vi "SplineHelp_ThomasAlgorithm.vi"(6 "inputSolutionVector":dbl[](array[numeric]), 8 "D":dbl[](array[numeric]), 9 "C":dbl[](array[numeric]), 10 "B":dbl[](array[numeric]), 11 "A":dbl[](array[numeric])) -> (0 "error out":errorcluster, 3 "SolutionVector":dbl[](array[numeric]))   [LabVIEW 2019, in "Trajectory_Library.lvlib"]
doc: "Thomas algorithm for solving tridiagonal systems Af = d.\n \nParameters:\n - a - the values of A above the diagonal\n - b - the values of A on the diagonal\n - c - the values of A below the diagonal\n - d - the vector on the rhs\n - InputSolutionVector - the unknown (solution) vector\n\nReturns:\n - SolutionVector - The modifed solution vector\n - Error Out - Returned error cluster"
uses:
  Trajectory_Library.lvlib
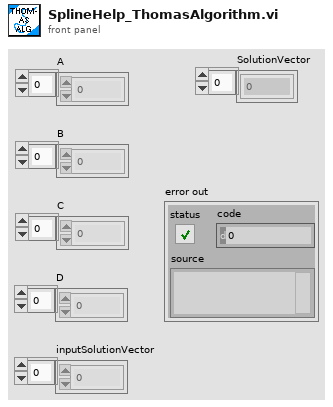
[diagram p1: front panel]
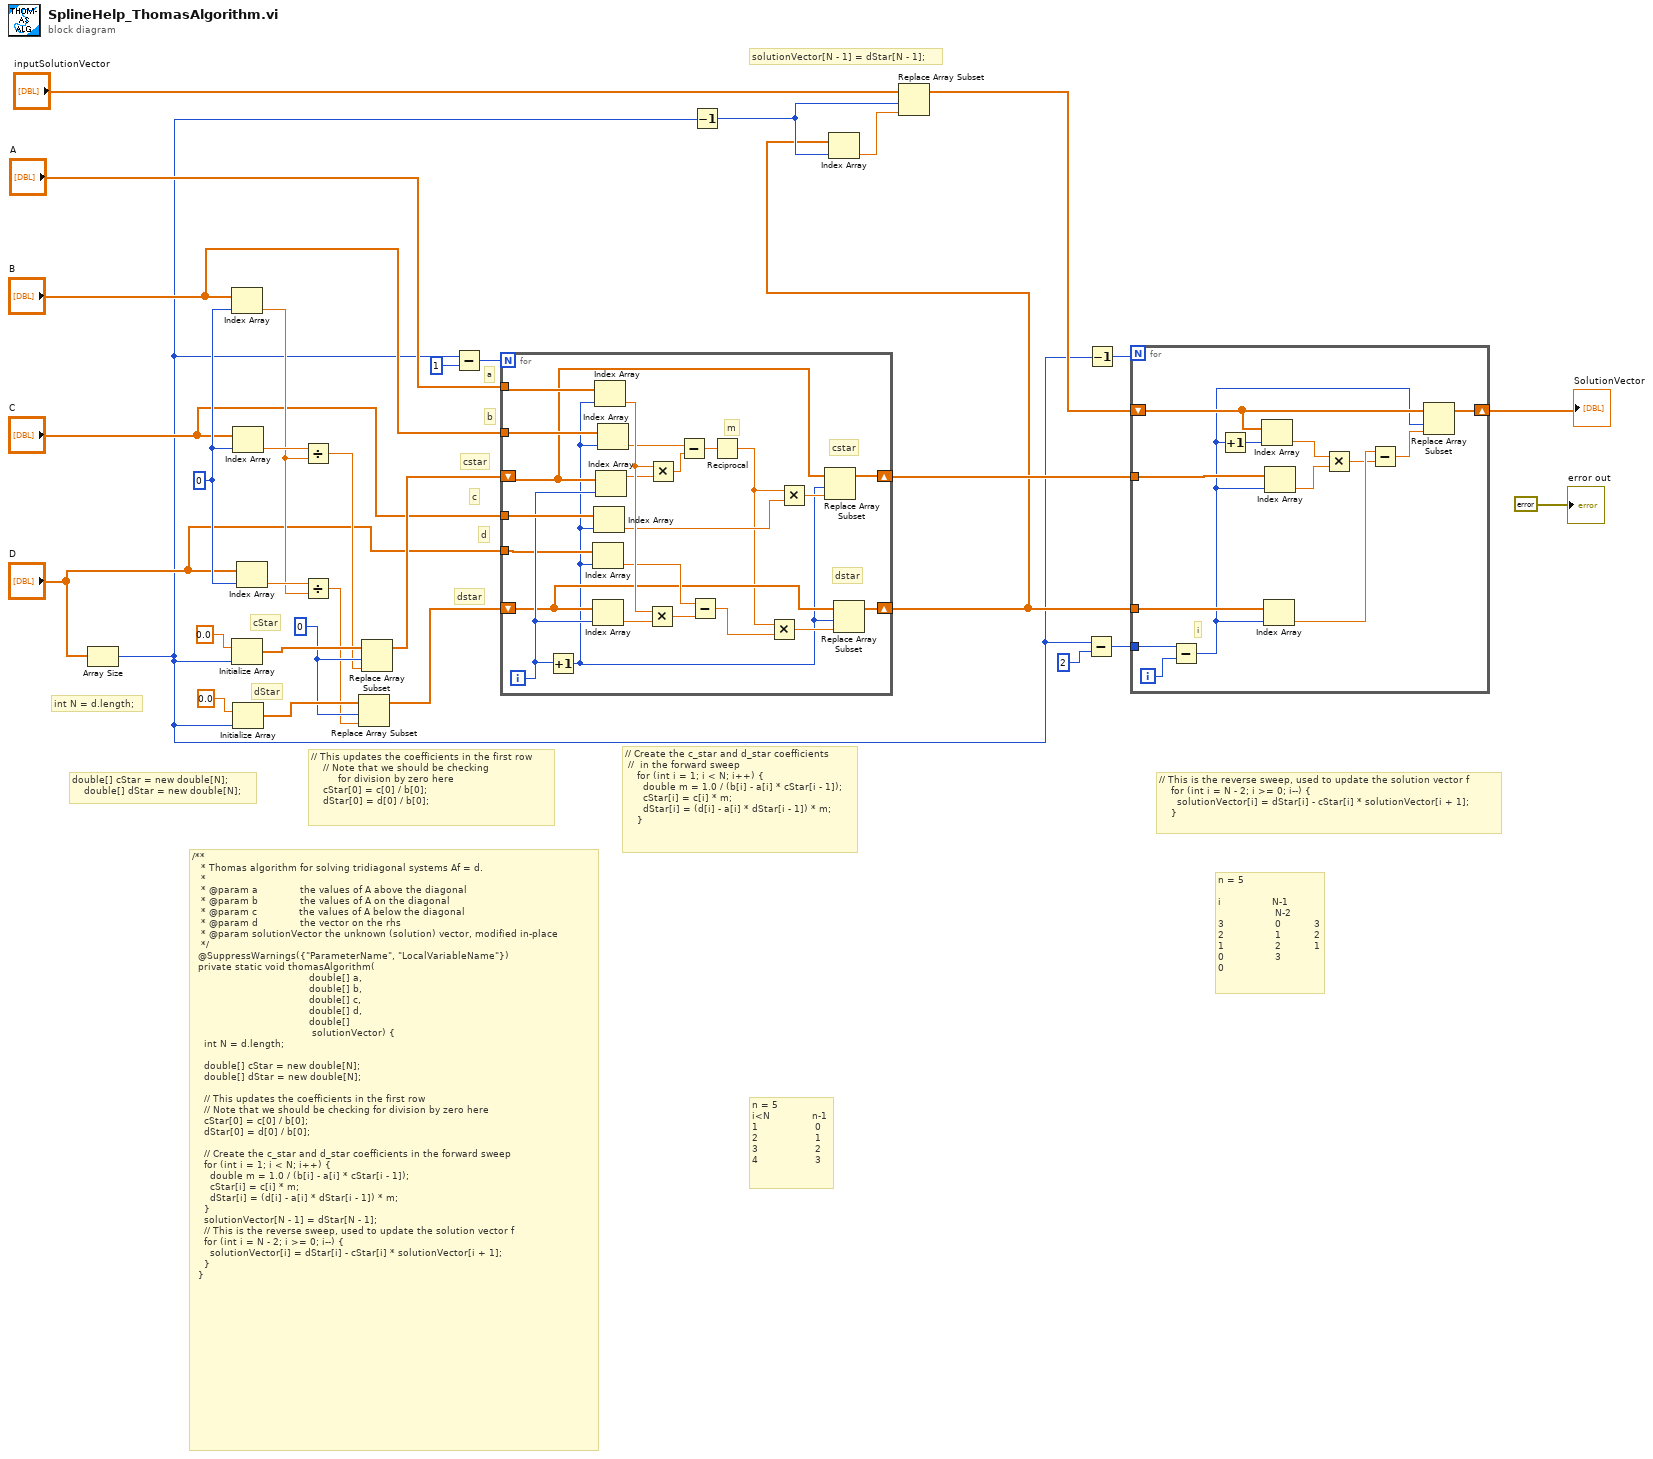
[diagram p0: block diagram]
diagram:
  w23 = 0 ("index")
  w29 = 0 ("index")
  # "n = 5\n\ni                 N-1\n                   N-2    \n3                 0           3\n2                 1           2\n1                 2           1\n0                 3            0"
  # "n = 5\ni<N              n-1\n1                   0\n2                   1\n3                   2\n4                   3"
  # "// This is the reverse sweep, used to update the solution vector f\n    for (int i = N - 2; i >= 0; i--) {\n      solutionVector[i] = dStar[i] - cStar[i] * solutionVector[i + 1];\n    }"
  # "solutionVector[N - 1] = dStar[N - 1];"
  # "d"
  # "dstar"
  # "c"
  # "cstar"
  # "b"
  # "a"
  # "// Create the c_star and d_star coefficients\n //  in the forward sweep\n    for (int i = 1; i < N; i++) {\n      double m = 1.0 / (b[i] - a[i] * cStar[i - 1]);\n      cStar[i] = c[i] * m;\n      dStar[i] = (d[i] - a[i] * dStar[i - 1]) * m;\n    }"
  # "// This updates the coefficients in the first row\n    // Note that we should be checking \n         for division by zero here\n    cStar[0] = c[0] / b[0];\n    dStar[0] = d[0] / b[0];"
  # "double[] cStar = new double[N];\n    double[] dStar = new double[N];"
  # "dStar"
  # "cStar"
  # "int N = d.length;"
  # "/**\n   * Thomas algorithm for solving tridiagonal systems Af = d.\n   *\n   * @param a              the values of A above the diagonal\n   * @param b              the values of A on the diagonal\n   * @param c              the values of A below the diagonal\n   * @param d              the vector on the rhs\n   * @param solutionVector the unknown (solution) vector, modified in-place\n   */\n  @SuppressWarnings({\"ParameterName\", \"LocalVariableName\"})\n  private static void thomasAlgorithm(\n                                       double[] a, \n                                       double[] b,\n                                       double[] c, \n                                       double[] d, \n                                       double[] \n                                        solutionVector) {\n    int N = d.length;\n\n    double[] cStar = new double[N];\n    double[] dStar = new double[N];\n\n    // This updates the coefficients in the first row\n    // Note that we should be checking for division by zero here\n    cStar[0] = c[0] / b[0];\n    dStar[0] = d[0] / b[0];\n\n    // Create the c_star and d_star coefficients in the forward sweep\n    for (int i = 1; i < N; i++) {\n      double m = 1.0 / (b[i] - a[i] * cStar[i - 1]);\n      cStar[i] = c[i] * m;\n      dStar[i] = (d[i] - a[i] * dStar[i - 1]) * m;\n    }\n    solutionVector[N - 1] = dStar[N - 1];\n    // This is the reverse sweep, used to update the solution vector f\n    for (int i = N - 2; i >= 0; i--) {\n      solutionVector[i] = dStar[i] - cStar[i] * solutionVector[i + 1];\n    }\n  }"
  n1 = Array Size(array="D") -> (size(s)=w2:i32)
  n2 = Index Array(array="B", index=w29) -> (element=w26:dbl)
  n3 = Initialize Array(0.0 ("element"), w2) -> (w25:dbl[])
  n4 = Index Array(array="C", index=w29) -> (element=w28:dbl)
  n5 = Initialize Array(0.0 ("element"), w2) -> (w24:dbl[])
  n6 = Index Array(array="D", index=w29) -> (element=w27:dbl)
  n7 = Divide(x=w28, y=w26) -> (x/y=w21:dbl)
  n8 = Divide(x=w27, y=w26) -> (x/y=w22:dbl)
  n9 = Replace Array Subset(array=w24, new element=w22, index=w23) -> (w18:dbl[])
  n10 = Replace Array Subset(array=w25, new element=w21, index=w23) -> (w19:dbl[])
  n11 = Subtract(x=w2, y=1) -> (x-y=w20:i32)
  n12 = for {
    N: w20 -> [_]
    tunnel: "A" -> [w54]
    tunnel: "B" -> [w52]
    tunnel: "C" -> [w49]
    shift-right: [w46] -> w7
    shift-left: w19 -> [w45]
    tunnel: "D" -> [w39]
    shift-right: [w36] -> w6
    shift-left: w18 -> [w35]
    i -> [w41]
    # "dstar"
    # "cstar"
    # "m"
    n13 = Increment(x=w41) -> (x+1=w32:i32)
    n14 = Index Array(array=w39, index=w32) -> (element=w38:dbl)
    n15 = Index Array(array=w35, index=w41) -> (element=w42:dbl)
    n16 = Index Array(array=w49, index=w32) -> (element=w43:dbl)
    n17 = Index Array(array=w54, index=w32) -> (element=w53:dbl)
    n18 = Index Array(array=w45, index=w41) -> (element=w47:dbl)
    n19 = Index Array(array=w52, index=w32) -> (element=w51:dbl)
    n20 = Multiply(x=w53, y=w42) -> (x*y=w40:dbl)
    n21 = Multiply(x=w53, y=w47) -> (x*y=w50:dbl)
    n22 = Subtract(x=w51, y=w50) -> (x-y=w48:dbl)
    n23 = Subtract(x=w38, y=w40) -> (x-y=w33:dbl)
    n24 = Reciprocal(x=w48) -> (1/x=w34:dbl)
    n25 = Multiply(x=w34, y=w33) -> (x*y=w37:dbl)
    n26 = Multiply(x=w34, y=w43) -> (x*y=w44:dbl)
    n27 = Replace Array Subset(array=w45, new element=w44, index=w32) -> (w46:dbl[])
    n28 = Replace Array Subset(array=w35, new element=w37, index=w32) -> (w36:dbl[])
  }
  n29 = Decrement(x=w2) -> (x-1=w12:i32)
  n30 = Index Array(array=w6, index=w12) -> (element=w11:dbl)
  n31 = Replace Array Subset(array="inputSolutionVector", new element=w11, index=w12) -> (w5:dbl[])
  n32 = Subtract(x=w2, y=2) -> (x-y=w9:i32)
  n33 = Decrement(x=w2) -> (x-1=w8:i32)
  n34 = for {
    N: w8 -> [_]
    tunnel: w9 -> [w66]
    tunnel: w7 -> [w64]
    tunnel: w6 -> [w63]
    shift-right: [w62] -> w4
    shift-left: w5 -> [w61]
    i -> [w67]
    # "i"
    n35 = Subtract(x=w66, y=w67) -> (x-y=w60:i32)
    n36 = Increment(x=w60) -> (x+1=w65:i32)
    n37 = Index Array(array=w61, index=w65) -> (element=w56:dbl)
    n38 = Index Array(array=w63, index=w60) -> (element=w58:dbl)
    n39 = Index Array(array=w64, index=w60) -> (element=w57:dbl)
    n40 = Multiply(x=w56, y=w57) -> (x*y=w55:dbl)
    n41 = Subtract(x=w58, y=w55) -> (x-y=w59:dbl)
    n42 = Replace Array Subset(array=w61, new element=w59, index=w60) -> (w62:dbl[])
  }
  "SolutionVector" <- w4
  "error out" <- errorcluster {"status"=FALSE, "code"=0, "source"=""} ("error constant")
